vi "sandbox.vi"() -> ()   [LabVIEW 2019]
uses:
  <userlib>/LevyLab/Transport/Control Experiment/Control Experiment.lvclass
  <userlib>/LevyLab/Instrument Framework/Instrument Types/Cryostat/Instrument.Cryostat.lvclass
panel:
  out "class name":string
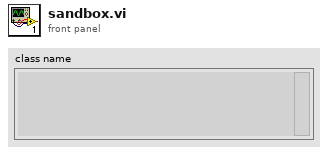
[diagram p1: front panel]
types:
  T1 = typedef "Control Experiment.lvclass/Instruments--cluster.ctl" = cluster{"KH7008":refnum<class "Instrument.KH7008.lvclass">[], "Lockin":refnum<class "Instrument.Lockin.lvclass">, "Temperature":refnum<class "Instrument.Cryostat.lvclass">, "Magnet":refnum<class "Instrument.Cryostat.lvclass">, "Rotator":refnum<class "Instrument.Cryostat.lvclass">, "Level":refnum<class "Instrument.Cryostat.lvclass">, "Capacitance Bridge":refnum<class "Instrument.CBridge.lvclass">, "Delay Line":refnum<class "Instrument.DelayLine.lvclass">, "Strain Cell":refnum<class "Instrument.Strain.lvclass">, "VNA":refnum<class "Instrument.VNA.lvclass">, "Voltage Source":refnum<class "Instrument.VSource.lvclass">}
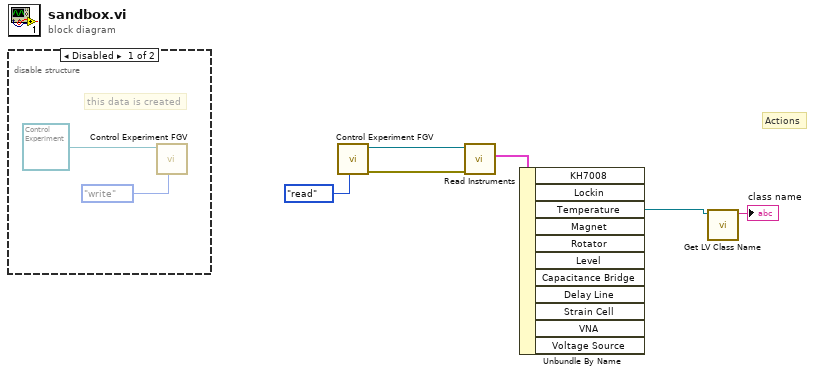
[diagram p0: block diagram]
diagram:
  # "Actions"
  n1 = disable-structure shown="Disabled" {
    frame Disabled {
      # "this data is created"
      n2 = call <userlib>:"Control Experiment FGV.vi"("Function"=enum16{"read", "write"}."write", "Control Experiment.lvclass"=refnum<class "Control Experiment.lvclass"> refnum) -> ()  [unwired: 8 in, 2 out]
    }
    frame Enabled {
    }
  }
  n3 = call <userlib>:"Control Experiment FGV.vi"("Function"=enum16{"read", "write"}."read") -> ("error out"=w4:errorcluster, "Control Experiment.lvclass out"=w5:refnum<class "Control Experiment.lvclass">)  [unwired: 9 in]
  n4 = call <userlib>:"Read Instruments.vi"("error in (no error)"=w4, "Control Experiment in"=w5) -> ("Instruments"=w3:T1)  [unwired: 7 in, 2 out]
  n5 = Unbundle By Name(w3) -> ("Temperature"=w2:refnum<class "Instrument.Cryostat.lvclass">)  [unwired: 10 out]
  n6 = call <vilib>:"Get LV Class Name.vi"("object"=w2) -> ("class name"=→"class name":string)  [unwired: 9 in, 1 out]
